vi "ImageFFTMasking.vi"(6 "shift?":bool=TRUE, 9 "Mask Percentage":dbl, 10 "Mask":dbl[][][](array[numeric]), 11 "Images":dbl[][][](array[numeric])) -> (2 "IFFTs":dbl[][][](array[numeric]), 3 "FFTs":dbl[][][](array[numeric]))   [LabVIEW 2012]
uses:
  <vilib>/Analysis/2dsp.llb/2D Real FFT.vi
  <vilib>/Analysis/2dsp.llb/2D Inverse Complex FFT.vi
  <vilib>/Analysis/NI_AALPro.lvlib
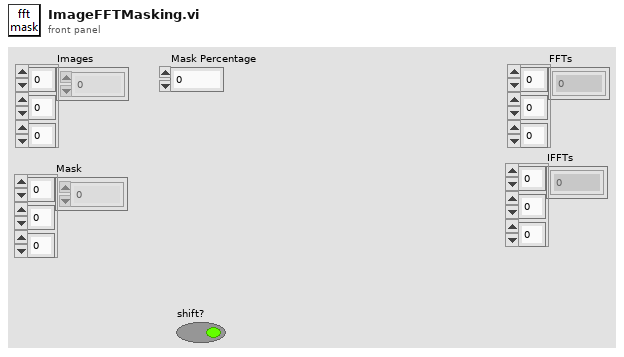
[diagram p1: front panel]
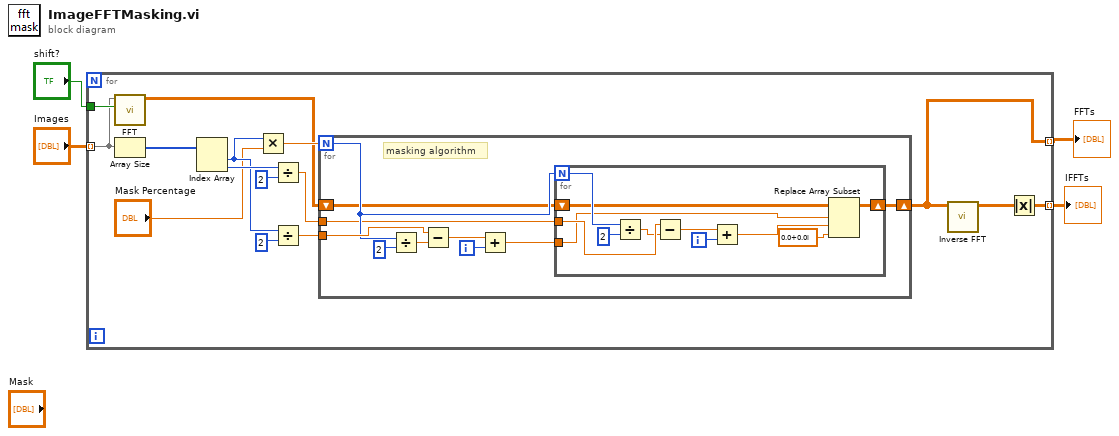
[diagram p0: block diagram]
diagram:
  n1 = for {
    tunnel: [w19] -> w2 mode=indexing
    tunnel: "shift?" -> [w17]
    tunnel: "Images" -> [w16] mode=indexing
    tunnel: [w5] -> w1 mode=indexing
    n2 = call-poly <vilib>:"FFT.vi"("shift?"=w17, "X"=w16) -> ("FFT {X}"=w6:cdb[][])  [unwired: 8 in, 1 out]
    n3 = Array Size(array=w16) -> (size(s)=w15:i32[])
    n4 = Index Array(array=w15) -> (element #1=w11:i32, element #2=w14:i32)  [unwired: 2 in]
    n5 = Multiply(x=w11, y="Mask Percentage") -> (x*y=w9:dbl)
    n6 = Divide(x=w14, y=2) -> (x/y=w7:dbl)
    n7 = Divide(x=w11, y=2) -> (x/y=w8:dbl)
    n8 = for {
      N: w9 -> [w24]
      tunnel: w8 -> [w27]
      tunnel: w7 -> [w23]
      shift-right: [w20] -> w5
      shift-left: w6 -> [w21]
      i -> [w25]
      # "masking algorithm"
      n9 = Divide(x=w24, y=2) -> (x/y=w28:dbl)
      n10 = Subtract(x=w27, y=w28) -> (x-y=w26:dbl)
      n11 = Add(x=w26, y=w25) -> (x+y=w22:dbl)
      n12 = for {
        N: w24 -> [w40]
        tunnel: w23 -> [w38]
        tunnel: w22 -> [w33]
        shift-right: [w31] -> w20
        shift-left: w21 -> [w32]
        i -> [w35]
        n13 = Divide(x=w40, y=2) -> (x/y=w37:dbl)
        n14 = Subtract(x=w38, y=w37) -> (x-y=w36:dbl)
        n15 = Add(x=w36, y=w35) -> (x+y=w34:dbl)
        n16 = Replace Array Subset(array=w32, new element=cdb 0.0+0.0i ("new element/subarray"), index (row)=w33, index (col)=w34) -> (w31:cdb[][])
      }
    }
    n17 = call-poly <vilib>:"Inverse FFT.vi"("FFT {x}"=w5) -> ("X"=w18:cdb[][])  [unwired: 9 in, 1 out]
    n18 = Absolute Value(x=w18) -> (abs(x)=w19:dbl[][])
  }
  "FFTs" <- w1
  "IFFTs" <- w2
